vi "Setup.vi"(8 "error in (no error)":errorcluster, 11 "Process Test In":refnum<class "Customer With Phone Test.lvclass">) -> (0 "error out":errorcluster, 3 "Process Test Out":refnum<class "Customer With Phone Test.lvclass">)   [LabVIEW 2020]
uses:
  <vilib>/Asteme/Triarc Framework Test Suite/Base Class Test/Base Test.lvclass
  Customer With Phone/Customer With Phone.lvclass
  Customer With Phone Test.lvclass
  C:/Program Files (x86)/National Instruments/LabVIEW 2020/vi.lib/Asteme/LUnit/Test Case.lvclass
  C:/Program Files (x86)/National Instruments/LabVIEW 2020/vi.lib/Asteme/Triarc Framework Test Suite/Base Class Test/Base Test.lvclass
  C:/Users/anton/Documents/GitHub/Triarc-Examples/Coffee Shop/Processes/People/Customers/Customer/Customer.lvclass
  C:/Users/anton/Documents/GitHub/Triarc-Examples/Coffee Shop/Processes/People/Person/Person.lvclass
  C:/Program Files (x86)/National Instruments/LabVIEW 2020/vi.lib/Asteme/Triarc Framework/View/View.lvclass
  C:/Program Files (x86)/National Instruments/LabVIEW 2020/vi.lib/Asteme/Triarc Framework/Process/Process.lvclass
  C:/Program Files (x86)/National Instruments/LabVIEW 2020/vi.lib/Asteme/Triarc Framework/Base/Base.lvclass
  C:/Program Files (x86)/National Instruments/LabVIEW 2020/vi.lib/Asteme/Triarc Framework/Error Handler Interface/Error Handler Interface.lvclass
  C:/Program Files (x86)/National Instruments/LabVIEW 2020/vi.lib/Asteme/Triarc Framework/Logging/Logging.lvclass
  C:/Users/anton/Documents/GitHub/Triarc-Examples/Coffee Shop/Processes/People/Process Job/Job Handler.lvclass
  C:/Program Files (x86)/National Instruments/LabVIEW 2020/vi.lib/Asteme/Triarc Framework/Asynchronous Action/Async Action.lvclass
  C:/Users/anton/Documents/GitHub/Triarc-Examples/Coffee Shop/Customer With Phone/Customer With Phone.lvclass
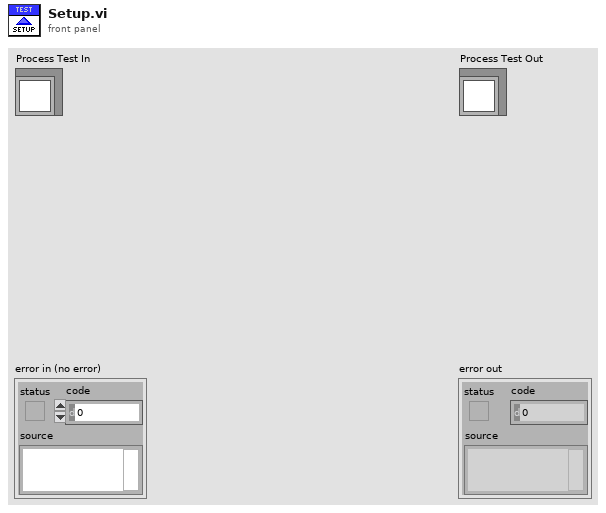
[diagram p1: front panel]
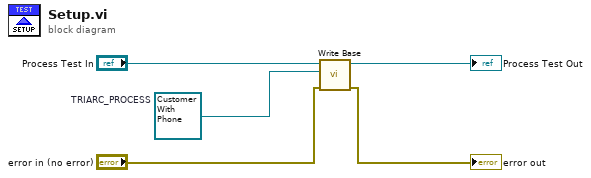
[diagram p0: block diagram]
diagram:
  w3 = refnum<class "Customer With Phone.lvclass"> refnum  # TRIARC_PROCESS
  n1 = call <vilib>:"Write Base.vi"("error in (no error)"="error in (no error)", "Base"=w3, "Base Class Test In"="Process Test In") -> ("error out"=→"error out":errorcluster, "Base Class Test Out"=→"Process Test Out":refnum<class "Base Test.lvclass">)  [unwired: 7 in]
